vi "TOSA_MCS_Switch.vi"() -> ()   [LabVIEW 2012]
uses:
  <vilib>/DAQmx/create/channels.llb/DAQmx Create Channel (CO-Pulse Generation-Ticks).vi
  <vilib>/DAQmx/configure/timing.llb/DAQmx Timing (Implicit).vi
  <resource>/objmgr/daqmx.rc
  <vilib>/DAQmx/create/channels.llb/DAQmx Create Channel (DO-Digital Output).vi
panel:
  out "Error Out":errorcluster
  in  "stop 3":bool
  in  "Error In 3":errorcluster
  out "Error Out 3":errorcluster
  in  "Error In":errorcluster
  in  "Stop":bool
  in  "pulse count":u32=150 min=4 max=9000 step=2
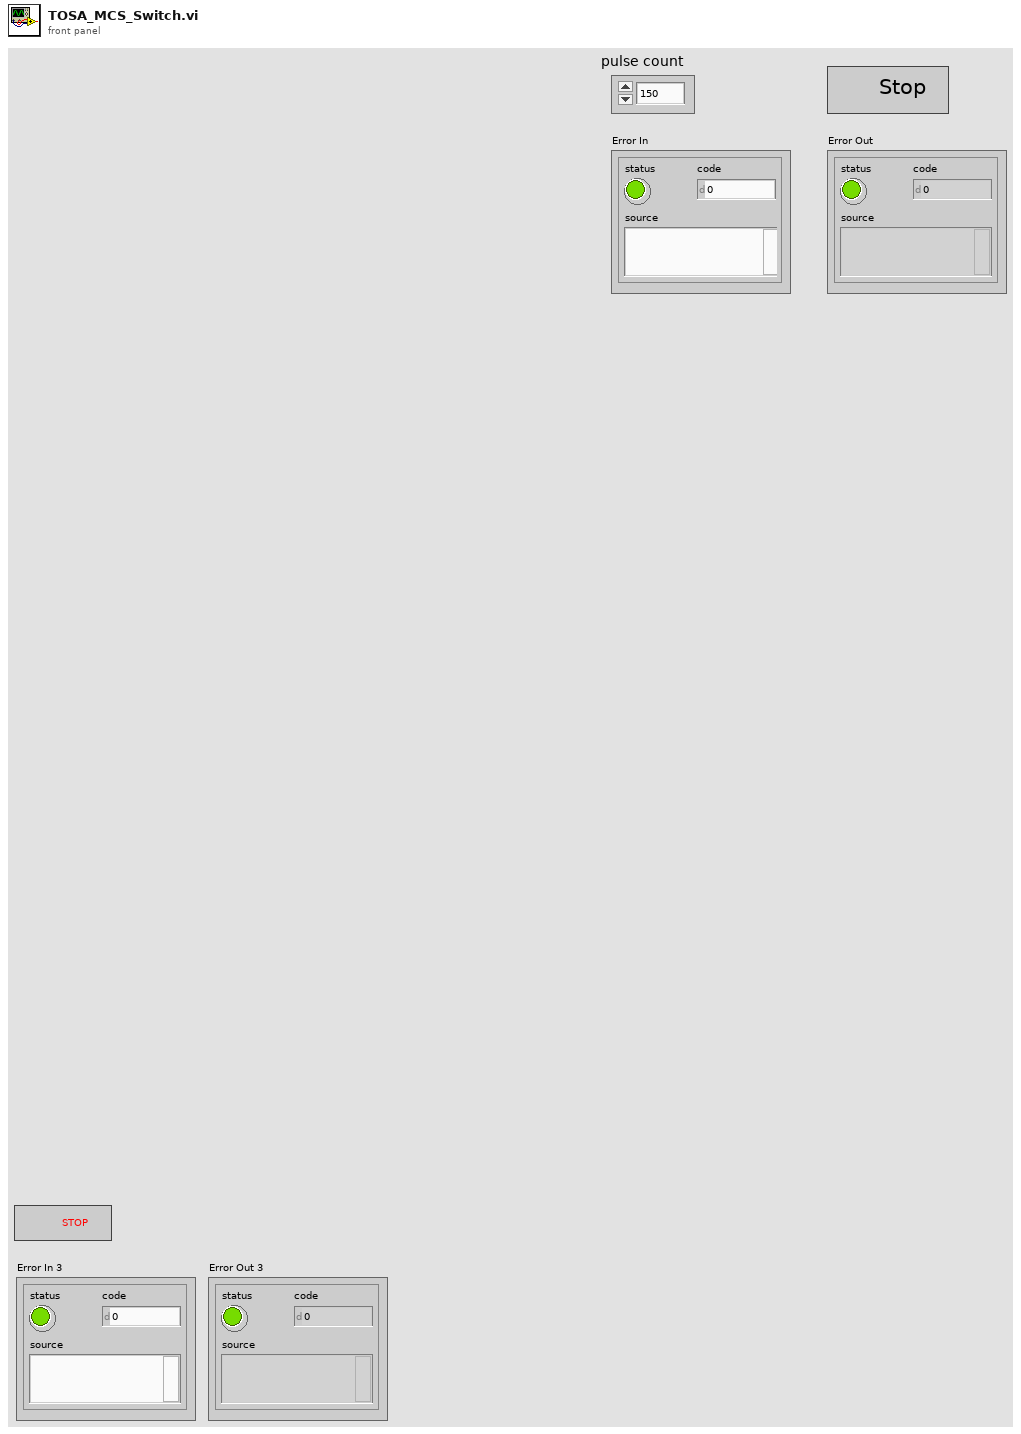
[diagram p1: front panel]
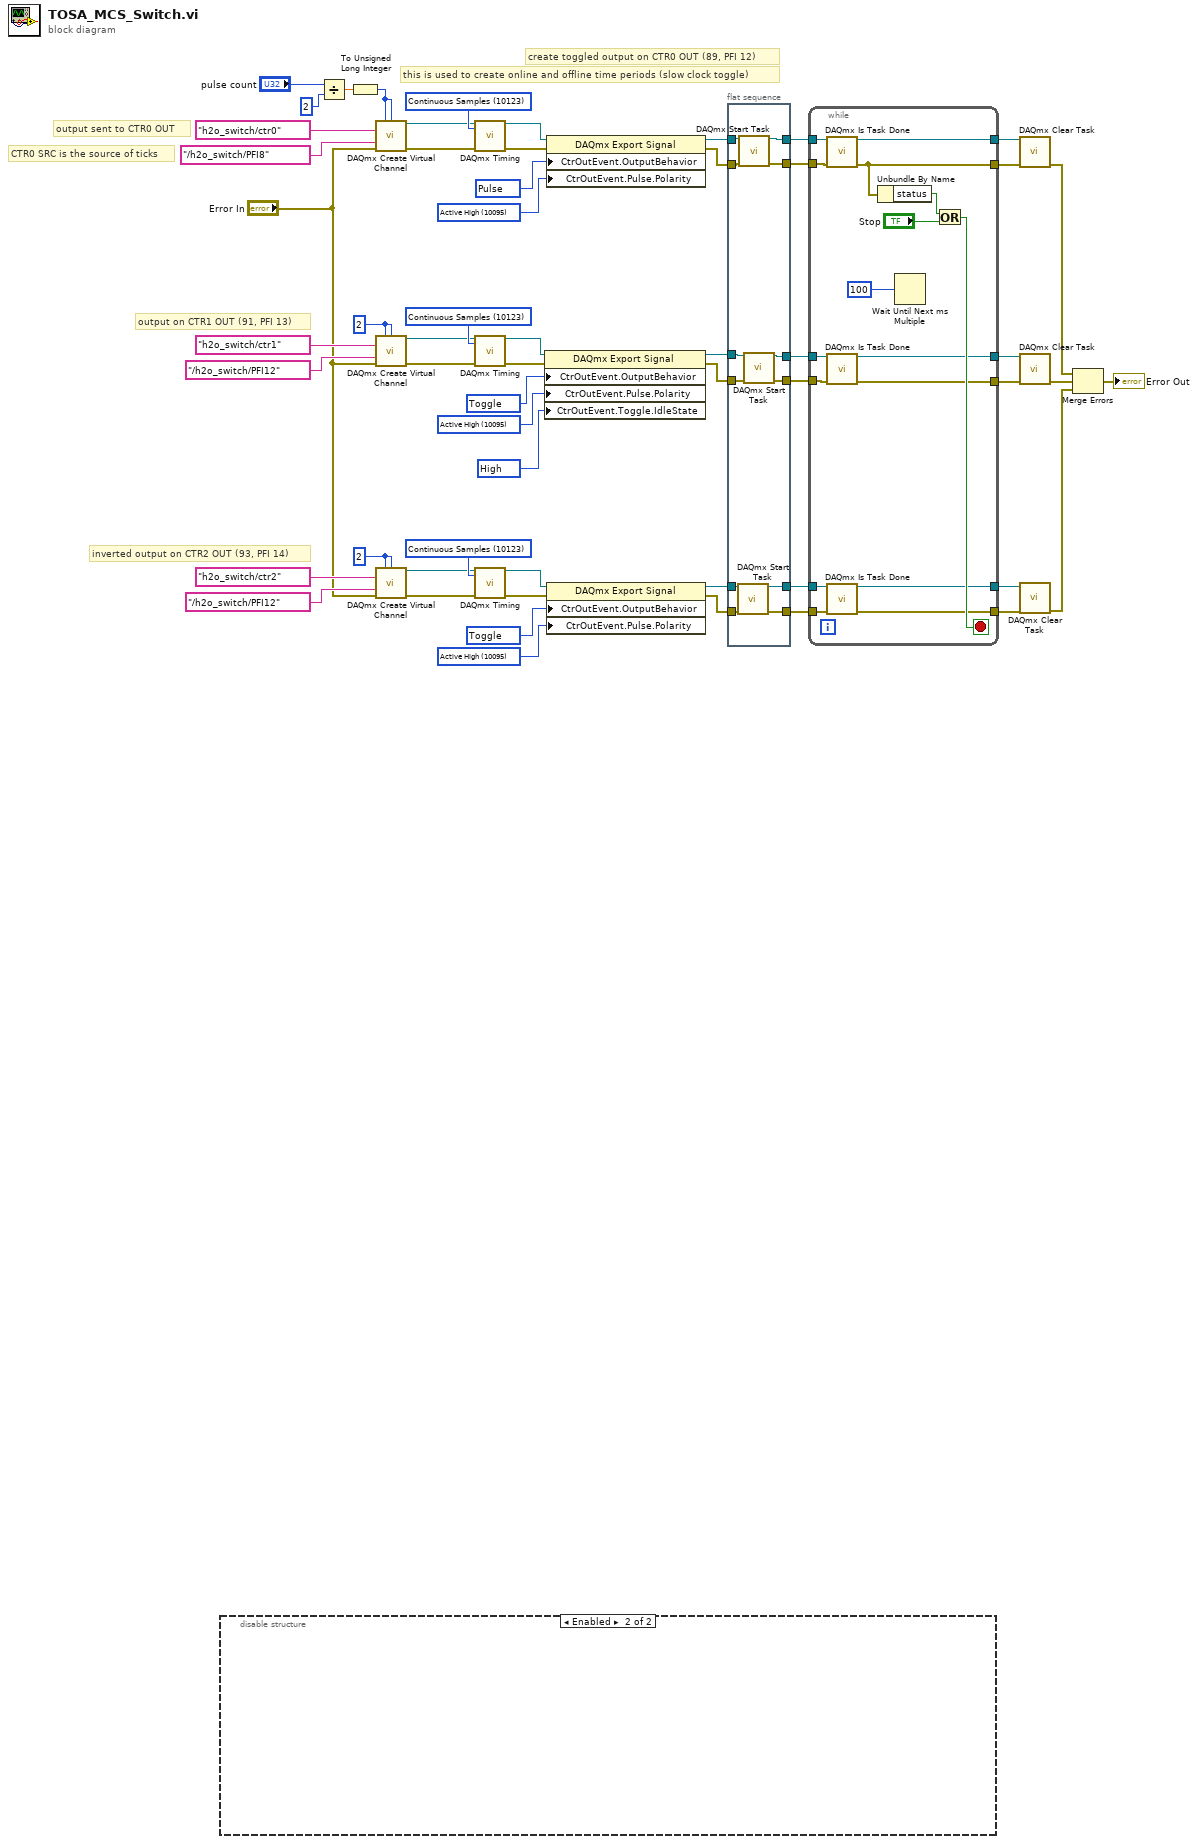
[diagram p0: block diagram]
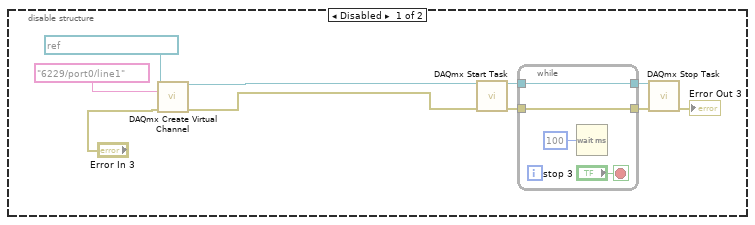
[diagram p2: hidden frame]
diagram:
  w9 = 10192 items=["High"=10192, "Low"=10214] ("CtrOutEvent.Toggle.IdleState")
  w17 = u32 2 ("high ticks")
  w20 = 10095 items=["Active High"=10095, "Active Low"=10096] ("CtrOutEvent.Pulse.Polarity")
  w26 = 10307 items=["Pulse"=10265, "Toggle"=10307] ("CtrOutEvent.OutputBehavior")
  w23 = 10123 items=["Finite Samples"=10178, "Continuous Samples"=10123, "Hardware Timed Single Point"=12522] ("sample mode")
  w27 = u32 2 ("high ticks")
  w38 = 10095 items=["Active High"=10095, "Active Low"=10096] ("CtrOutEvent.Pulse.Polarity")
  w44 = 10307 items=["Pulse"=10265, "Toggle"=10307] ("CtrOutEvent.OutputBehavior")
  w41 = 10123 items=["Finite Samples"=10178, "Continuous Samples"=10123, "Hardware Timed Single Point"=12522] ("sample mode")
  w45 = 10095 items=["Active High"=10095, "Active Low"=10096] ("CtrOutEvent.Pulse.Polarity")
  w57 = 10265 items=["Pulse"=10265, "Toggle"=10307] ("CtrOutEvent.OutputBehavior")
  w49 = 10123 items=["Finite Samples"=10178, "Continuous Samples"=10123, "Hardware Timed Single Point"=12522] ("sample mode")
  # "inverted output on CTR2 OUT (93, PFI 14)"
  # "output on CTR1 OUT (91, PFI 13)"
  # "output sent to CTR0 OUT"
  # "CTR0 SRC is the source of ticks"
  # "this is used to create online and offline time periods (slow clock toggle)"
  # "create toggled output on CTR0 OUT (89, PFI 12)"
  n1 = disable-structure shown="Enabled" {
    frame Disabled {
      n2 = call-poly <vilib>:"DAQmx Create Virtual Channel.vi"("task in"=refnum<k21> "MyDigitalOutTask_0", "lines"=tag "6229/port0/line1", "error in"="Error In 3") -> ("task out"=w60:refnum<k21>, "error out"=w59:errorcluster)  [unwired: 11 in]
      n3 = call <vilib>:"DAQmx Start Task.vi"("task/channels in"=w60, "error in"=w59) -> ("task out"=w63:refnum<k21>, "error out"=w64:errorcluster)  [unwired: 12 in]
      n4 = while {
        tunnel: w63 -> [w69]
        tunnel: w64 -> [w68]
        tunnel: [w69] -> w67
        tunnel: [w68] -> w66
        stop <- "stop 3" stop-if-true
        n5 = Wait (ms)(milliseconds to wait=u32 100) -> ()  [unwired: 1 out]
      }
      n6 = call <vilib>:"DAQmx Stop Task.vi"("task/channels in"=w67, "error in"=w66) -> ("error out"=→"Error Out 3":errorcluster)  [unwired: 12 in, 1 out]
    }
    frame Enabled {
    }
  }
  n7 = Divide(x="pulse count", y=u32 2) -> (x/y=w7:dbl)
  n8 = To Unsigned Long Integer(number=w7) -> (unsigned 32bit integer=w5:u32)
  n9 = call-poly <vilib>:"DAQmx Create Virtual Channel.vi"("high ticks"=w5, "low ticks"=w5, "counter"=tag "h2o_switch/ctr0", "source of ticks"=tag "/h2o_switch/PFI8", "error in"="Error In") -> ("task out"=w47:refnum<k21>, "error out"=w48:errorcluster)  [unwired: 9 in]
  n10 = call-poly <vilib>:"DAQmx Create Virtual Channel.vi"("high ticks"=w27, "low ticks"=w27, "counter"=tag "h2o_switch/ctr1", "source of ticks"=tag "/h2o_switch/PFI12", "error in"="Error In") -> ("task out"=w39:refnum<k21>, "error out"=w40:errorcluster)  [unwired: 9 in]
  n11 = call-poly <vilib>:"DAQmx Create Virtual Channel.vi"("high ticks"=w17, "low ticks"=w17, "counter"=tag "h2o_switch/ctr2", "source of ticks"=tag "/h2o_switch/PFI12", "error in"="Error In") -> ("task out"=w21:refnum<k21>, "error out"=w22:errorcluster)  [unwired: 9 in]
  n12 = call-poly <vilib>:"DAQmx Timing.vi"("task/channels in"=w47, "sample mode"=w49, "error in"=w48) -> ("task out"=w55:refnum<k21>, "error out"=w53:errorcluster)  [unwired: 11 in]
  n13 = call-poly <vilib>:"DAQmx Timing.vi"("task/channels in"=w39, "sample mode"=w41, "error in"=w40) -> ("task out"=w43:refnum<k21>, "error out"=w42:errorcluster)  [unwired: 11 in]
  n14 = call-poly <vilib>:"DAQmx Timing.vi"("task/channels in"=w21, "sample mode"=w23, "error in"=w22) -> ("task out"=w25:refnum<k21>, "error out"=w24:errorcluster)  [unwired: 11 in]
  n15 = property class="DAQmx Export Signal"(reference=w43, error in=w42, "CtrOutEvent.OutputBehavior"=w44, "CtrOutEvent.Pulse.Polarity"=w38, "CtrOutEvent.Toggle.IdleState"=w9) -> (reference out=w36:refnum<k21>, error out=w34:errorcluster)
  n16 = property class="DAQmx Export Signal"(reference=w55, error in=w53, "CtrOutEvent.OutputBehavior"=w57, "CtrOutEvent.Pulse.Polarity"=w45) -> (reference out=w56:refnum<k21>, error out=w54:errorcluster)
  n17 = property class="DAQmx Export Signal"(reference=w25, error in=w24, "CtrOutEvent.OutputBehavior"=w26, "CtrOutEvent.Pulse.Polarity"=w20) -> (reference out=w15:refnum<k21>, error out=w14:errorcluster)
  n18 = flat-sequence {
    tunnel: [w81] -> w50
    tunnel: [w80] -> w46
    tunnel: [w78] -> w35
    tunnel: [w76] -> w33
    tunnel: [w73] -> w13
    tunnel: [w72] -> w12
    tunnel: w56 -> [w82]
    tunnel: w54 -> [w83]
    tunnel: w36 -> [w79]
    tunnel: w34 -> [w77]
    tunnel: w15 -> [w75]
    tunnel: w14 -> [w74]
    frame #0 {
      n19 = call <vilib>:"DAQmx Start Task.vi"("task/channels in"=w75, "error in"=w74) -> ("task out"=w73:refnum<k21>, "error out"=w72:errorcluster)  [unwired: 12 in]
      n20 = call <vilib>:"DAQmx Start Task.vi"("task/channels in"=w82, "error in"=w83) -> ("task out"=w81:refnum<k21>, "error out"=w80:errorcluster)  [unwired: 12 in]
      n21 = call <vilib>:"DAQmx Start Task.vi"("task/channels in"=w79, "error in"=w77) -> ("task out"=w78:refnum<k21>, "error out"=w76:errorcluster)  [unwired: 12 in]
    }
  }
  n22 = while {
    tunnel: w50 -> [w99]
    tunnel: w46 -> [w98]
    tunnel: [w95] -> w52
    tunnel: [w96] -> w51
    tunnel: w35 -> [w88]
    tunnel: w33 -> [w89]
    tunnel: [w91] -> w32
    tunnel: [w90] -> w31
    tunnel: w13 -> [w87]
    tunnel: w12 -> [w86]
    tunnel: [w85] -> w11
    tunnel: [w84] -> w10
    stop <- w97 stop-if-true
    n23 = call <vilib>:"DAQmx Is Task Done.vi"("task/channels in"=w99, "error in"=w98) -> ("task out"=w96:refnum<k21>, "error out"=w95:errorcluster)  [unwired: 11 in, 1 out]
    n24 = call <vilib>:"DAQmx Is Task Done.vi"("task/channels in"=w88, "error in"=w89) -> ("task out"=w91:refnum<k21>, "error out"=w90:errorcluster)  [unwired: 11 in, 1 out]
    n25 = call <vilib>:"DAQmx Is Task Done.vi"("task/channels in"=w87, "error in"=w86) -> ("task out"=w85:refnum<k21>, "error out"=w84:errorcluster)  [unwired: 11 in, 1 out]
    n26 = Unbundle By Name(w95) -> ("status"=w94:bool)
    n27 = Wait Until Next ms Multiple(millisecond multiple=u32 100) -> ()  [unwired: 1 out]
    n28 = Or(x=w94, y="Stop") -> (x .or. y?=w97:bool)
  }
  n29 = call <vilib>:"DAQmx Clear Task.vi"("task in"=w51, "error in"=w52) -> ("error out"=w4:errorcluster)  [unwired: 13 in]
  n30 = call <vilib>:"DAQmx Clear Task.vi"("task in"=w32, "error in"=w31) -> ("error out"=w3:errorcluster)  [unwired: 13 in]
  n31 = call <vilib>:"DAQmx Clear Task.vi"("task in"=w11, "error in"=w10) -> ("error out"=w2:errorcluster)  [unwired: 13 in]
  n32 = Merge Errors(w4, w3, w2) -> (→"Error Out":errorcluster)
